vi "Apply.vi"(8 "error in (no error)":errorcluster, 9 "Fs (Hz)":dbl, 10 "Array in":dbl[](array[numeric]), 11 "SAM in":refnum<class "SAM.lvclass">) -> (0 "error out":errorcluster, 2 "Array out":dbl[](array[numeric]), 3 "SAM out":refnum<class "SAM.lvclass">)   [LabVIEW 2020, in "SAM.lvclass"]
uses:
  SAM.lvclass
  D:/Development/epl-vi-lib/Signal Synthesis VIs/4th Generation/Classes/Modulations/AM/AM.lvclass
  SAM.lvclass/SAM.ctl
  AM/AM.lvclass/AM.ctl
  AM/Read Depth (0-1).vi
  <vilib>/Analysis/NI_AALBase.lvlib
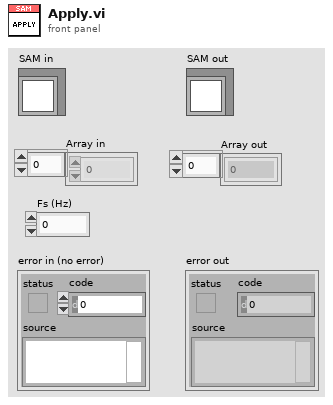
[diagram p1: front panel]
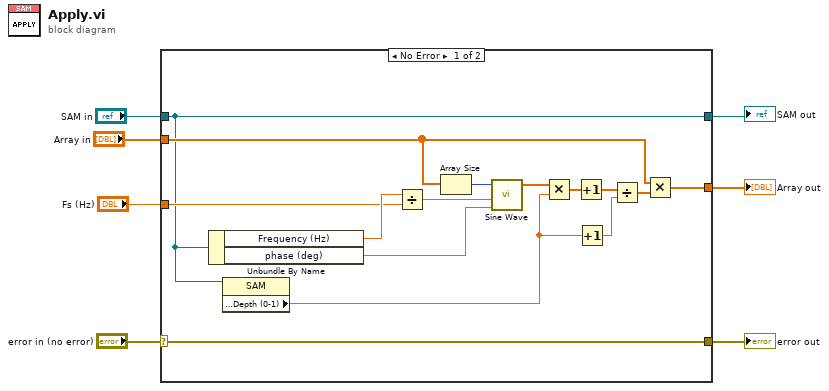
[diagram p0: block diagram]
diagram:
  n1 = case shown="No Error" "error in (no error)" {
    selector: "error in (no error)" -> [w22 w25]
    tunnel: [w22 w25] -> w1
    tunnel: "Fs (Hz)" -> [w14 _]
    tunnel: [w11 w23] -> w4
    tunnel: "SAM in" -> [w9 w24]
    tunnel: [w9 w24] -> w5
    tunnel: "Array in" -> [w10 w23]
    frame No Error {
      n2 = Unbundle By Name(w9) -> ("Frequency (Hz)"=w21:dbl, "phase (deg)"=w13:dbl)
      n3 = property class="SAM"(reference=w9) -> ("Accessors:Depth (0-1)"=w8:dbl)  [unwired: 1 in, 2 out]
      n4 = Divide(x=w21, y=w14) -> (x/y=w20:dbl)
      n5 = Array Size(array=w10) -> (size(s)=w15:i32)
      n6 = call <vilib>:"Sine Wave.vi"("samples"=w15, "frequency"=w20, "phase in"=w13) -> ("sine wave"=w19:dbl[])  [unwired: 2 in, 2 out]
      n7 = Multiply(x=w19, y=w8) -> (x*y=w18:dbl[])
      n8 = Increment(x=w18) -> (x+1=w17:dbl[])
      n9 = Increment(x=w8) -> (x+1=w16:dbl)
      n10 = Divide(x=w17, y=w16) -> (x/y=w12:dbl[])
      n11 = Multiply(x=w10, y=w12) -> (x*y=w11:dbl[])
    }
    frame Error {
    }
  }
  "error out" <- w1
  "SAM out" <- w5
  "Array out" <- w4
